vi "NewSnake.vi"(8 "error in (no error)":errorcluster, 11 "SnakeData1":T1) -> (0 "error out":errorcluster, 3 "Snake out":refnum<class "Snake.lvclass">)   [LabVIEW 2019, in "RT_Game.lvlib" / "Snake.lvclass"]
uses:
  Snake.lvclass
  SnakeGame/SnakeData.ctl
  SnakeGame/Direction.ctl
  Game/Coordinate.ctl
  SnakeGame/CoordinateData.ctl
  Snake.lvclass/Snake.ctl
  SnakeGame/SnakeGame.lvclass
  Game/Game.lvclass
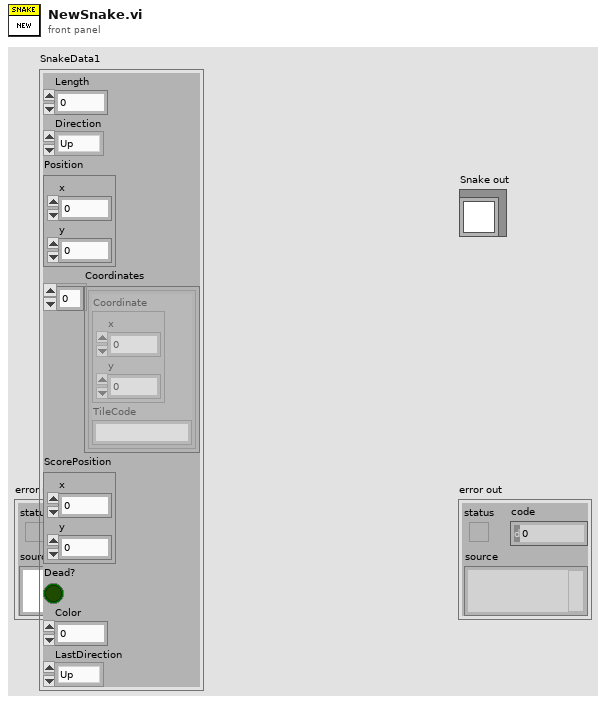
[diagram p1: front panel]
types:
  T1 = typedef "RT_Game.lvlib/SnakeGame.lvclass/SnakeData.ctl" = cluster{"Length":i16, "Direction":T2, "Position":T3, "Coordinates":T4[], "ScorePosition":T3, "Dead?":bool, "Color":fxp<+,3,3>, "LastDirection":T2}
  T2 = typedef "RT_Game.lvlib/SnakeGame.lvclass/Direction.ctl" = enum16{"Up", "Left", "Down", "Right"}
  T3 = typedef "RT_Game.lvlib/Game.lvclass/Coordinate.ctl" = cluster{"x":dbl, "y":dbl}
  T4 = typedef "RT_Game.lvlib/SnakeGame.lvclass/CoordinateData.ctl" = cluster{"Coordinate":T3, "TileCode":string}
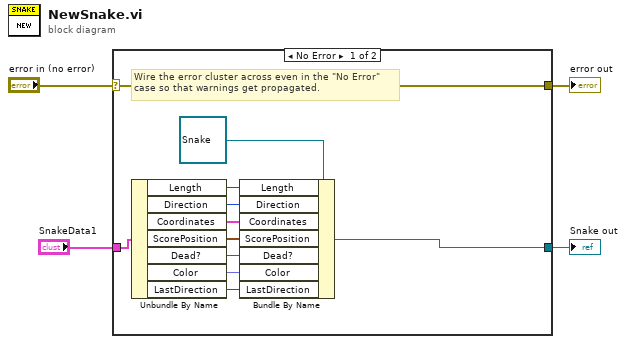
[diagram p0: block diagram]
diagram:
  n1 = case shown="No Error" "error in (no error)" {
    selector: "error in (no error)" -> [w15 w16]
    tunnel: [w15 w16] -> w3
    tunnel: [w12 _] -> w2
    tunnel: "SnakeData1" -> [w13 _]
    frame No Error {
      # "Wire the error cluster across even in the \"No Error\"\ncase so that warnings get propagated."
      n2 = Unbundle By Name(w13) -> ("Length"=w11:i16, "Direction"=w10:T2, "Coordinates"=w9:T4[], "ScorePosition"=w8:T3, "Dead?"=w7:bool, "Color"=w6:fxp<+,3,3>, "LastDirection"=w5:T2)
      n3 = Bundle By Name(cluster=refnum<class "Snake.lvclass"> refnum ("Snake out"), "Length"=w11, "Direction"=w10, "Coordinates"=w9, "ScorePosition"=w8, "Dead?"=w7, "Color"=w6, "LastDirection"=w5) -> (w12:refnum<class "Snake.lvclass">)
    }
    frame Error {
    }
  }
  "error out" <- w3
  "Snake out" <- w2
